vi "view_all_4_peaks.vi"(1 "activity":dbl[][](array[numeric])) -> (0 "Cluster":T1)   [LabVIEW 2009]
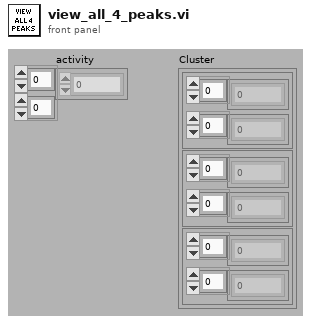
[diagram p1: front panel]
types:
  T1 = cluster{cluster{dbl[], dbl[]}, cluster{dbl[], dbl[]}, cluster{dbl[], dbl[]}}
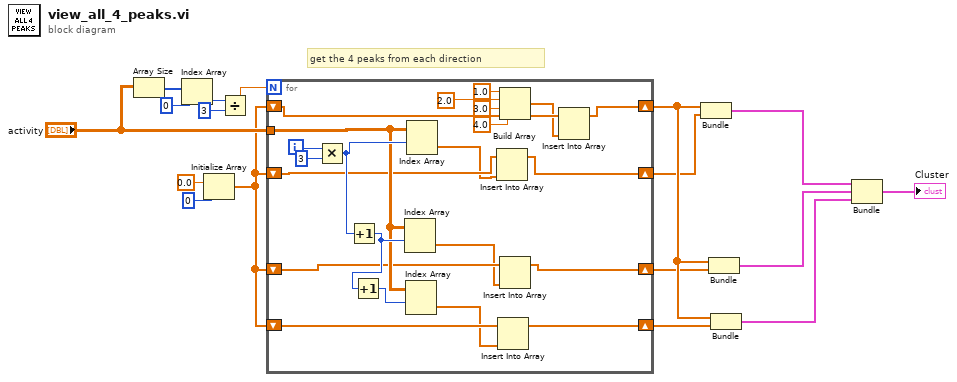
[diagram p0: block diagram]
diagram:
  # "get the 4 peaks from each direction"
  n1 = Array Size(array="activity") -> (size(s)=w1:i32[])
  n2 = Index Array(array=w1, index=0) -> (element=w3:i32)
  n3 = Initialize Array(0.0 ("element"), 0 ("dimension size")) -> (w8:dbl[])
  n4 = Divide(x=w3, y=3) -> (x/y=w5:dbl)
  n5 = for {
    N: w5 -> [_]
    tunnel: "activity" -> [w34]
    shift-right: [w31] -> w9
    shift-left: w8 -> [w33]
    shift-right: [w28] -> w10
    shift-left: w8 -> [w30]
    shift-right: [w25] -> w11
    shift-left: w8 -> [w27]
    shift-right: [w20] -> w12
    shift-left: w8 -> [w22]
    i -> [w39]
    n6 = Multiply(x=w39, y=3) -> (x*y=w37:i32)
    n7 = Increment(x=w37) -> (x+1=w36:i32)
    n8 = Increment(x=w36) -> (x+1=w35:i32)
    n9 = Index Array(array=w34, index (row)=w36) -> (element=w29:dbl[])  [unwired: 1 in]
    n10 = Index Array(array=w34, index (row)=w35) -> (element=w26:dbl[])  [unwired: 1 in]
    n11 = Index Array(array=w34, index (row)=w37) -> (element=w32:dbl[])  [unwired: 1 in]
    n12 = Insert Into Array(array=w33, new element=w32) -> (w31:dbl[])  [unwired: 1 in]
    n13 = Insert Into Array(array=w27, new element=w26) -> (w25:dbl[])  [unwired: 1 in]
    n14 = Build Array(1.0 ("element"), 2.0 ("element"), 3.0 ("element"), 4.0 ("element")) -> (w21:dbl[])
    n15 = Insert Into Array(array=w30, new element=w29) -> (w28:dbl[])  [unwired: 1 in]
    n16 = Insert Into Array(array=w22, new element=w21) -> (w20:dbl[])  [unwired: 1 in]
  }
  n17 = Bundle(w12, w9) -> (w14:cluster{dbl[], dbl[]})  [unwired: 1 in]
  n18 = Bundle(w12, w10) -> (w15:cluster{dbl[], dbl[]})  [unwired: 1 in]
  n19 = Bundle(w12, w11) -> (w16:cluster{dbl[], dbl[]})  [unwired: 1 in]
  n20 = Bundle(w14, w15, w16) -> (→"Cluster":T1)  [unwired: 1 in]
